vi "Run Simulator VI.vi"(8 "error in (no error)":errorcluster, 11 "TCS in":refnum<class "TCS.lvclass">) -> (0 "error out":errorcluster, 3 "TCS out":refnum<class "TCS.lvclass">)   [LabVIEW 2018, in "TCS.lvclass"]
uses:
  TCS.lvclass
  TCS.lvclass/TCS.ctl
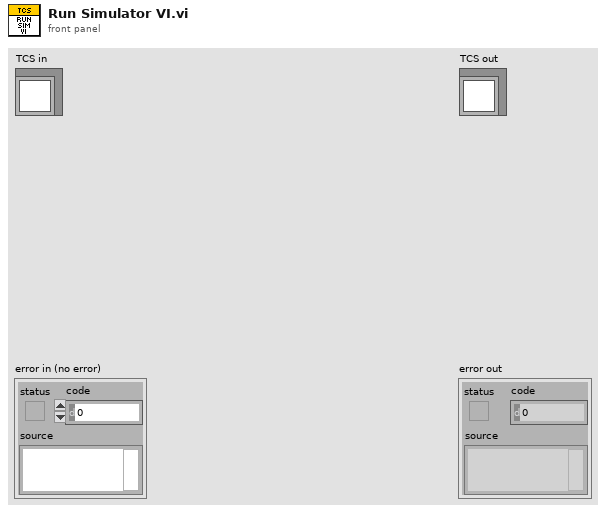
[diagram p1: front panel]
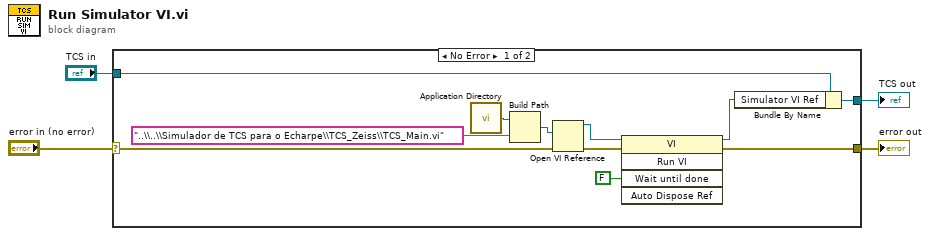
[diagram p0: block diagram]
diagram:
  n1 = case shown="No Error" "error in (no error)" {
    selector: "error in (no error)" -> [w12 w17]
    tunnel: [w10 w17] -> w3
    tunnel: [w7 w16] -> w1
    tunnel: "TCS in" -> [w9 w16]
    frame No Error {
      n2 = call <vilib>:"Application Directory.vi"() -> ("Application Directory"=w15:path)
      n3 = Build Path(base path=w15, name or relative path="..\\..\\Simulador de TCS para o Echarpe\\TCS_Zeiss\\TCS_Main.vi") -> (appended path=w13:path)
      n4 = Open VI Reference(vi path=w13, error in (no error)=w12) -> (vi reference=w6:refnum<vi>, error out=w5:errorcluster)  [unwired: 4 in]
      n5 = invoke class="VI" method="Run VI"(reference=w6, error in=w5, "Wait until done"=FALSE ("Wait Until Done")) -> (reference out=w8:refnum<vi>, error out=w10:errorcluster)  [unwired: 2 in, 3 out]
      n6 = Bundle By Name(cluster=w9, "Simulator VI Ref"=w8) -> (w7:refnum<class "TCS.lvclass">)
    }
    frame Error {
    }
  }
  "error out" <- w3
  "TCS out" <- w1
